vi "CS-4 Read Mag Current.vi"(3 "error in (no error)":errorcluster, 5 "VISA session":refnum<visa-resource-name>) -> (0 "error out":errorcluster, 1 "response out":string, 2 "dup VISA session":refnum<visa-resource-name>)   [LabVIEW 2016]
doc: "CS-4 Read Current.vi will return the present supply output current reading."
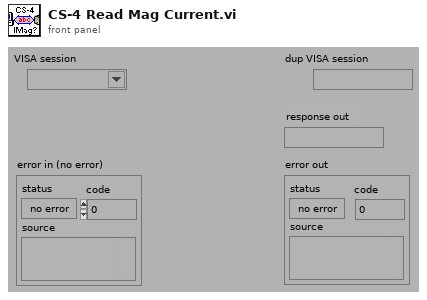
[diagram p1: front panel]
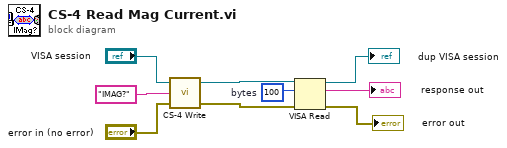
[diagram p0: block diagram]
diagram:
  w3 = u32 100  # bytes
  n1 = call "CS-4 Write.vi"("error in (no error)"="error in (no error)", "write buffer (\"\")"="IMAG?", "VISA session"="VISA session") -> ("error out"=w6:errorcluster, "dup VISA session"=w7:refnum<visa-resource-name>)  [unwired: 1 out]
  n2 = VISA Read(VISA resource name=w7, byte count=w3, error in (no error)=w6) -> (VISA resource name out=→"dup VISA session":refnum<visa-resource-name>, read buffer=→"response out":string, error out=→"error out":errorcluster)  [unwired: 1 out]
